vi "SignRec7265ReadX.vi"(2 "Point #":i32, 3 "Instrument Address":refnum<visa-resource-name>) -> (0 "Stop":bool, 1 "Measurement":dbl[](array[numeric]) format="%.6e")   [LabVIEW 2025]
doc: "This VI reads a single X reading from a Signal Recovery 7265 Lock IN. The stop boolean is always false. If no reading is obtained a single zero is returned.\n NHMFL-FSU, Jan 2008\nAuthor: Scott Hannahs <sth@magnet.fsu.edu>\n\nThis software is licensed for use under the “MIT License\"\nCopyright (c) 2025 Scott Hannahs, sth@sth@magnet.sthnet.net\n\nPermission is hereby granted, free of charge, to any person obtaining a copy of this software and associated documentation files (the \"Software\"), to deal in the Software without restriction, including without limitation the rights to use, copy, modify, merge, publish, distribute, sublicense, and/or sell copies of the Software, and to permit persons to whom the Software is furnished to do so, subject to the following conditions: The above copyright notice and this permission notice shall be included in all copies or substantial portions of the Software.\n\nTHE SOFTWARE IS PROVIDED \"AS IS\", WITHOUT WARRANTY OF ANY KIND, EXPRESS OR IMPLIED, INCLUDING BUT NOT LIMITED TO THE WARRANTIES OF MERCHANTABILITY, FITNESS FOR A PARTICULAR PURPOSE AND NONINFRINGEMENT. IN NO EVENT SHALL THE AUTHORS OR COPYRIGHT HOLDERS BE LIABLE FOR ANY CLAIM, DAMAGES OR OTHER LIABILITY, WHETHER IN AN ACTION OF CONTRACT, TORT OR OTHERWISE, ARISING FROM, OUT OF OR IN CONNECTION WITH THE SOFTWARE OR THE USE OR OTHER DEALINGS IN THE SOFTWARE."
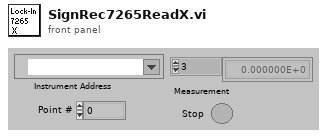
[diagram p1: front panel]
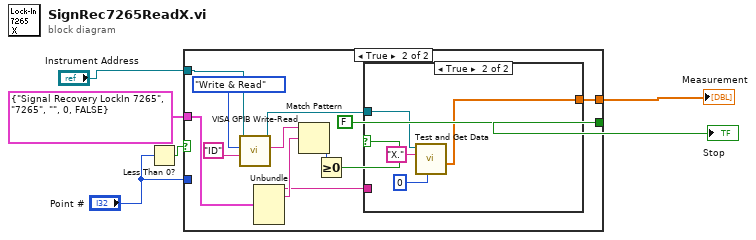
[diagram p0: block diagram]
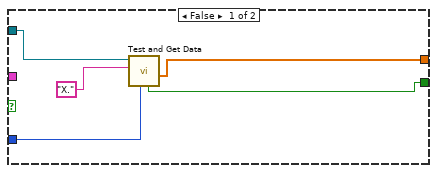
[diagram p2: hidden frame]
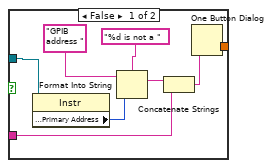
[diagram p3: hidden frame]
diagram:
  n1 = Less Than 0?(x="Point #") -> (x < 0?=w5:bool)
  n2 = case shown="True" w5 {
    tunnel: cluster{string, string, string, u32, bool} {"Signal Recovery LockIn 7265", "7265", "", 0, FALSE} -> [_ w15]
    tunnel: "Instrument Address" -> [w9 w23]
    tunnel: [w10 FALSE ("Stop")] -> w3
    tunnel: [w11 w12] -> w2
    tunnel: "Point #" -> [w8 _]
    frame False {
      n3 = call "Test and Get Data.vi"("Point #"=w8, "Command String"="X.", "VISA Sesson"=w9) -> ("Measurement"=w11:dbl[], "Stop"=w10:bool)  [unwired: 3 in, 3 out]
    }
    frame True {
      n4 = call "VISA GPIB Write-Read.vi"("Command"="ID", "Action"=enum16{"Write", "Read", "Write & Read"}."Write & Read", "VISA resource name"=w23) -> ("String Returned"=w19:string, "dup VISA Session"=w20:refnum<visa-resource-name>)  [unwired: 5 in, 2 out]
      n5 = Unbundle(w15) -> (w14:string, w16:string)  [unwired: 3 out]
      n6 = Match Pattern(string=w19, regular expression=w16) -> (offset past match=w18:i32)  [unwired: 1 in, 3 out]
      n7 = Greater Or Equal To 0?(x=w18) -> (x >= 0?=w17:bool)
      n8 = case shown="True" w17 {
        tunnel: w20 -> [w26 w31]
        tunnel: w14 -> [w24 _]
        tunnel: [_ w32] -> w12
        frame False {
          n9 = property class="Instr"(reference=w26) -> ("GPIB Settings:Primary Address"=w25:u16)  [unwired: 1 in, 2 out]
          n10 = Format Into String(format string="%d is not a ", initial string="GPIB address ", w25) -> (resulting string=w30:string)  [unwired: 1 in, 1 out]
          n11 = Concatenate Strings(w30, w24) -> (w27:string)
          n12 = One Button Dialog(message=w27) -> ()  [unwired: 1 in, 1 out]
        }
        frame True {
          n13 = call "Test and Get Data.vi"("Point #"=0, "Command String"="X.", "VISA Sesson"=w31) -> ("Measurement"=w32:dbl[])  [unwired: 3 in, 4 out]
        }
      }
    }
  }
  "Measurement" <- w2
  "Stop" <- w3
